vi "Can send requests.vi"(8 "error in (no error)":errorcluster, 9 "Topic URI":string, 10 "Serialisation":T1, 11 "WAMP Client in":refnum<class "WAMP Client.lvclass">) -> (0 "error out":errorcluster, 3 "WAMP Client out":refnum<class "WAMP Client.lvclass">)   [LabVIEW 2020, in "wamplv.lvlib" / "WAMP Client.lvclass"]
uses:
  WAMP Client.lvclass
  WAMP Client.lvclass/WAMP Client.ctl
  API/TypeDefs/Serialisation.ctl
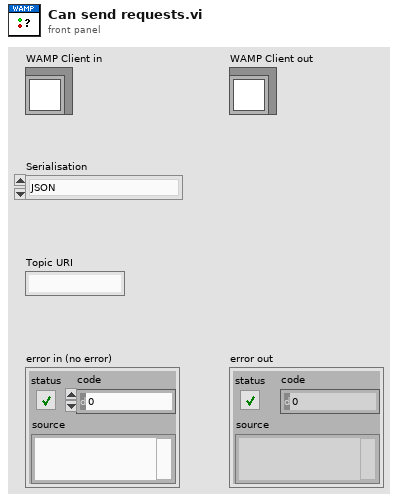
[diagram p1: front panel]
types:
  T1 = typedef "wamplv.lvlib/WAMP Client.lvclass/Serialisation.ctl" = enum16{"JSON", "MessagePack"}
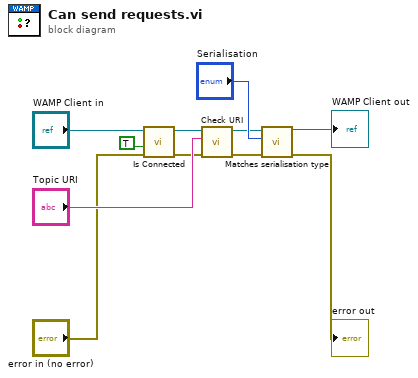
[diagram p0: block diagram]
diagram:
  n1 = call "Is Connected.vi"("error in"="error in (no error)", "Raise error if not connected"=TRUE, "WAMP Client in"="WAMP Client in") -> ("error out"=w3:errorcluster, "WAMP Client out"=w5:refnum<class "WAMP Client.lvclass">)  [unwired: 6 in, 1 out]
  n2 = call "Check URI.vi"("error in (no error)"=w3, "URI"="Topic URI", "WAMP Client in"=w5) -> ("error out"=w8:errorcluster, "WAMP Client out"=w7:refnum<class "WAMP Client.lvclass">)  [unwired: 5 in, 2 out]
  n3 = call "Matches serialisation type.vi"("error in (no error)"=w8, "Serialisation"="Serialisation", "WAMP Client in"=w7) -> ("error out"=→"error out":errorcluster, "WAMP Client out"=→"WAMP Client out":refnum<class "WAMP Client.lvclass">)  [unwired: 6 in, 1 out]
